vi "33-Update Trace Data.vi"(8 "error in":errorcluster, 10 "Over":bool, 11 "S6F1":T1) -> (0 "error out":errorcluster)   [LabVIEW 2020, in "SECS Scenarios.lvlib" / "Scenarios Class.lvclass"]
uses:
  Scenarios Class.lvclass
  SECS Communication/S6 Message Class/S6F1.ctl
  33-Update Trace Data.ctl
  SECS Communication/SECS-II Class/Format Code.ctl
  SECS Communication/SECS-II Class/SECS-II Class.lvclass
  SECS Communication/S6 Message Class/S6 Message Class.lvclass
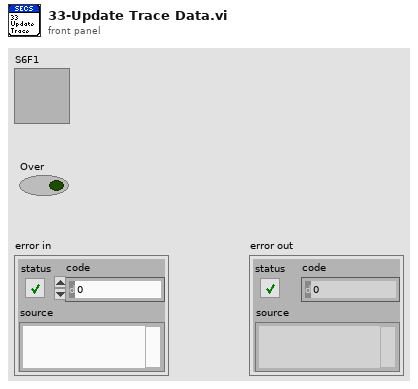
[diagram p1: front panel]
types:
  T1 = typedef "SECS Communication.lvlib/S6 Message Class.lvclass/S6F1.ctl" = cluster{"TRID":u32, "SMPLN":u32, "STIME":string, "SV":cluster{"Format Code":T2, "Value":variant}[]}
  T2 = typedef "SECS Communication.lvlib/SECS-II Class.lvclass/Format Code.ctl" = enum16{"L", "A", "B", "Boolean", "J", "I1", "I2", "I4", "I8", "U1", "U2", "U4", "U8", "F4", "F8", "Char"}
  T3 = typedef "SECS Scenarios.lvlib/Scenarios Class.lvclass/33-Update Trace Data.ctl" = cluster{"S6F1":T1, "Over":bool}
  T4 = typedef "SECS Scenarios.lvlib/Scenarios Class.lvclass/Request Refnum.ctl" = cluster{"11-Alarm Management":refnum<user-event>, "07-Event Report From Equipment":refnum<user-event>, "14-Process Program Creating Editing or Deleting":refnum<user-event>, "21-Material Movement":refnum<user-event>, "23-Equipment Sends Information to Host":refnum<user-event>, "24-Host Accepts On-Line Request from Equipment":refnum<user-event>, "25-Host Refuses On-Line Request":refnum<user-event>, "29-Equipment Requests Time Value from Host":refnum<user-event>, "33-Update Trace Data":refnum<user-event>}
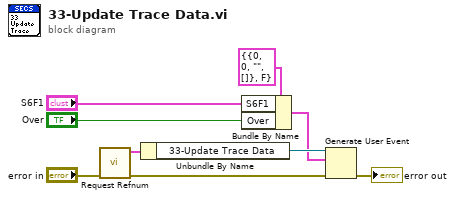
[diagram p0: block diagram]
diagram:
  n1 = call "Request Refnum.vi"("error in"="error in") -> ("error out"=w8:errorcluster, "Request Refnum"=w9:T4)  [unwired: 9 in]
  n2 = Unbundle By Name(w9) -> ("33-Update Trace Data"=w7:refnum<user-event>)
  n3 = Bundle By Name(cluster=T3 {"S6F1"={"TRID"=0, "SMPLN"=0, "STIME"="", "SV"=[]}, "Over"=FALSE} ("33-Update Trace Data"), "S6F1"="S6F1", "Over"="Over") -> (w6:T3)
  n4 = Generate User Event(user event=w7, event data cluster=w6, error in=w8) -> (error out=→"error out":errorcluster)  [unwired: 1 in, 1 out]
